vi "Chat (OpenAI).vi"(0 "Refnum in":T1, 1 "OpenAI-Compatible LLM URL":string, 5 "LLM Model Name":string, 7 "System Prompt":string, 9 "User Prompt":string, 11 "error in":errorcluster, 12 "reasoning":T2={"effort"=enum."low", "exclude"=FALSE}, 13 "Temperature":dbl=0.8) -> (4 "Refnum out":T1, 6 "previous messages":T3[](array[typedef]), 8 "Answer content":string, 10 "reasoning content":string, 15 "error out":errorcluster)   [LabVIEW 2023, in "LabVIEW LLM.lvlib"]
uses:
  LabVIEW LLM.lvlib
  openai_message.ctl
  <vilib>/httpClient/ClientHandle.ctl
  chat-completion req.ctl
  labview-ai-share/AI Base Globals.vi
  labview-ai-share/LabVIEW AI Base.lvlib
  <vilib>/httpClient/LabVIEWHTTPClient.lvlib
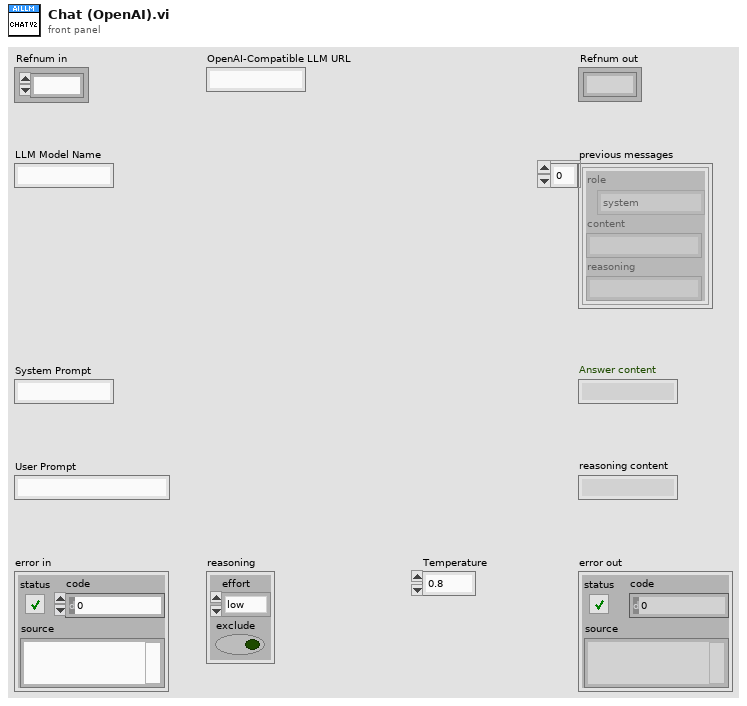
[diagram p1: front panel]
types:
  T1 = typedef "LabVIEWHTTPClient.lvlib/ClientHandle.ctl" = refnum<k1>
  T2 = cluster{"effort":enum16{"high", "medium", "low"}, "exclude":bool}
  T3 = typedef "LabVIEW LLM.lvlib/openai_message.ctl" = cluster{"role":enum16{"system", "user", "assistant"}, "content":string, "reasoning":string}
  T4 = typedef "LabVIEW LLM.lvlib/chat-completion req.ctl" = cluster{"model":string, "messages":T3[], "max_tokens":u32, "temperature":dbl, "stream":bool, "reasoning":cluster{"effort":enum16{"high", "medium", "low"}, "exclude":bool}}
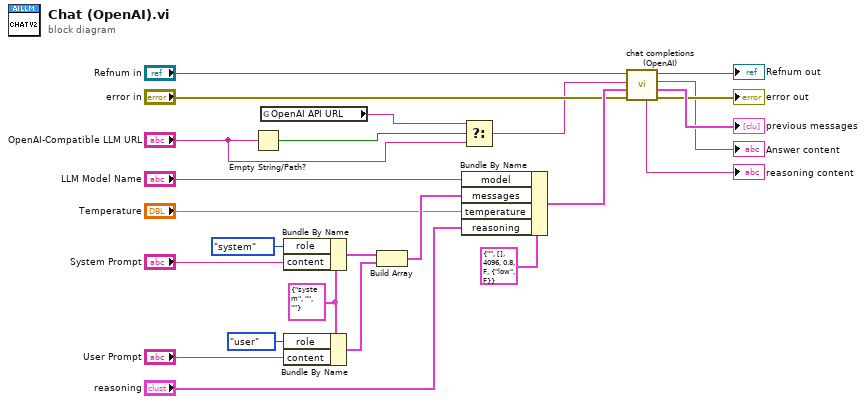
[diagram p0: block diagram]
diagram:
  w21 = T3 {"role"=enum."system", "content"="", "reasoning"=""} ("message")
  n1 = Empty String/Path?(string/path="OpenAI-Compatible LLM URL") -> (empty?=w4:bool)
  n2 = global read "AI Base Globals.vi" "OpenAI API URL"() -> (w6:string)
  n3 = Bundle By Name(cluster=w21, "role"=enum16{"system", "user", "assistant"}."system", "content"="System Prompt") -> (w14:T3)
  n4 = Bundle By Name(cluster=w21, "role"=enum16{"system", "user", "assistant"}."user", "content"="User Prompt") -> (w17:T3)
  n5 = Build Array(w14, w17) -> (w13:T3[])
  n6 = Bundle By Name(cluster=T4 {"model"="", "messages"=[], "max_tokens"=4096, "temperature"=0.8, "stream"=FALSE, "reasoning"={"effort"=enum."low", "exclude"=FALSE}}, "model"="LLM Model Name", "messages"=w13, "temperature"="Temperature", "reasoning"="reasoning") -> (w10:T4)
  n7 = Select(t=w6, s=w4, f="OpenAI-Compatible LLM URL") -> (s? t:f=w5:string)
  n8 = call "chat completions (OpenAI).vi"("error in"="error in", "chat-completion req"=w10, "API url"=w5, "Refnum in"="Refnum in") -> ("error out"=→"error out":errorcluster, "previous messages"=→"previous messages":T3[], "Answer content"=→"Answer content":string, "Refnum out"=→"Refnum out":T1, "reasoning content"=→"reasoning content":string)  [unwired: 3 in]
